vi "Update Action Status.vi"(5 "Data (orig)":path, 6 "Action in":T1, 9 "Data":path, 10 "Path Selector":refnum<class "MGI Path Selector.lvclass">, 11 "Path Selector (orig)":refnum<class "MGI Path Selector.lvclass">) -> (2 "State Change?":bool, 4 "Action out":T1)   [LabVIEW 2016, in "MGI Path Selector.lvclass"]
doc: "Update Action cluster if the specified data or class have changed.\n\nAuthored by Shawn Walpole\nsupport@mooregoodideas.com\nwww.mooregoodideas.com\n\nCopyright (c) 2013, Moore Good Ideas, Inc.\n\nAll rights reserved.\n\nRedistribution and use in source and binary forms, with or without modification, are permitted provided that the following conditions are met:\n\n * Redistributions of source code must retain the above copyright notice, this list of conditions and the following disclaimer.\n * Redistributions in binary form must reproduce the above copyright notice, this list of conditions and the following disclaimer in the documentation and/or other materials provided with the distribution.\n * Neither the name of Moore Good Ideas, Inc. nor the names of its contributors may be used to endorse or promote products derived from this software without specific prior written permission.\n\nTHIS SOFTWARE IS PROVIDED BY THE COPYRIGHT HOLDERS AND CONTRIBUTORS \"AS IS\" AND ANY EXPRESS OR IMPLIED WARRANTIES, INCLUDING, BUT NOT LIMITED TO, THE IMPLIED WARRANTIES OF MERCHANTABILITY AND FITNESS FOR A PARTICULAR PURPOSE ARE DISCLAIMED. IN NO EVENT SHALL THE COPYRIGHT OWNER OR CONTRIBUTORS BE LIABLE FOR ANY DIRECT, INDIRECT, INCIDENTAL, SPECIAL, EXEMPLARY, OR CONSEQUENTIAL DAMAGES (INCLUDING, BUT NOT LIMITED TO, PROCUREMENT OF SUBSTITUTE GOODS OR SERVICES; LOSS OF USE, DATA, OR PROFITS; OR BUSINESS INTERRUPTION) HOWEVER CAUSED AND ON ANY THEORY OF LIABILITY, WHETHER IN CONTRACT, STRICT LIABILITY, OR TORT (INCLUDING NEGLIGENCE OR OTHERWISE) ARISING IN ANY WAY OUT OF THE USE OF THIS SOFTWARE, EVEN IF ADVISED OF THE POSSIBILITY OF SUCH DAMAGE."
uses:
  <userlib>/_MGI/User Interface/Path Selector XControl/Class Hierarchy/MGI Path Selector.lvclass
  <vilib>/_xctls/Action.ctl
  <vilib>/_xctls/XControlSupport.lvlib
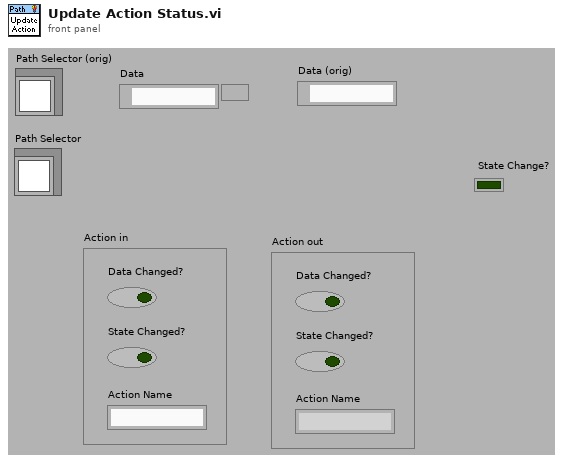
[diagram p1: front panel]
types:
  T1 = typedef "XControlSupport.lvlib/Action.ctl" = cluster{"Data Changed?":bool, "State Changed?":bool, "Action Name":string}
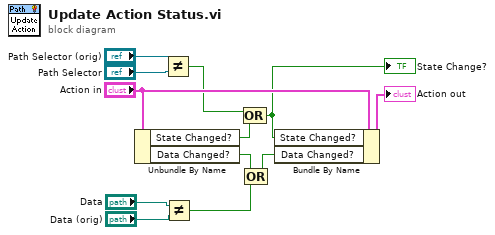
[diagram p0: block diagram]
diagram:
  n1 = Unbundle By Name("Action in") -> ("State Changed?"=w9:bool, "Data Changed?"=w6:bool)
  n2 = Not Equal?(x="Path Selector (orig)", y="Path Selector") -> (x != y?=w8:bool)
  n3 = Not Equal?(x="Data", y="Data (orig)") -> (x != y?=w2:bool)
  n4 = Compound Arithmetic op=OR(w8, w9) -> (w1:bool)
  "State Change?" <- w1
  n5 = Compound Arithmetic op=OR(w6, w2) -> (w5:bool)
  n6 = Bundle By Name(cluster="Action in", "State Changed?"=w1, "Data Changed?"=w5) -> (→"Action out":T1)
